vi "Reset Window.vi"(8 "error in (no error)":errorcluster, 11 "Rigol DG822 Sine in":refnum<class "Rigol DG822 Sine.lvclass">) -> (0 "error out":errorcluster, 3 "Rigol DG822 Sine out":refnum<class "Rigol DG822 Sine.lvclass">)   [LabVIEW 2021, in "Rigol DG822 UI.lvlib" / "Rigol DG822 Sine.lvlib" / "Rigol DG822 Sine.lvclass"]
uses:
  Rigol DG822 Sine.lvclass
  General/Files/lvlibp/Actors.lvlibp/Actors/Actors/Actors.lvclass
  D:/LabVIEW/General/Files/lvlibp/Actors.lvlibp/Actors/Actors/Actors.lvclass
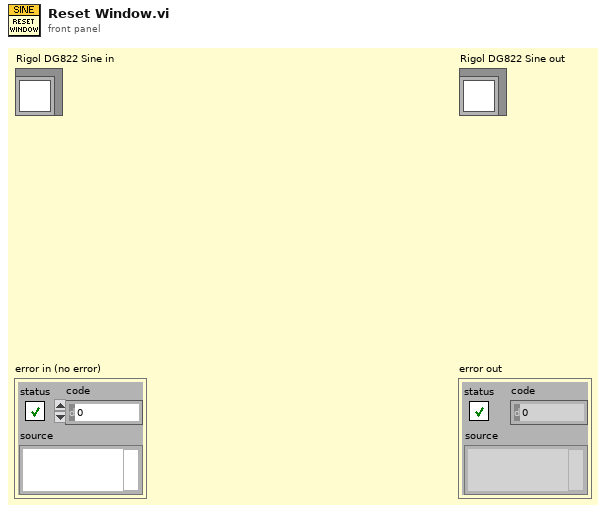
[diagram p1: front panel]
types:
  T1 = cluster{"Control Label 5":string, "Control Label 6":string, "Control Label":string, "Control Label 2":string, "Control Label 3":string, "Control Label 4":string}
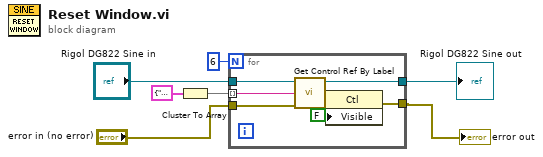
[diagram p0: block diagram]
diagram:
  n1 = Cluster To Array(cluster=T1 {"Control Label 5"="FreqUnit", "Control Label 6"="PeriodUnit", "Control Label"="AmplUnit", "Control Label 2"="HighLUnit", "Control Label 3"="OffsetUnit", "Control Label 4"="LowLUnit"}) -> (array=w6:string[])
  n2 = for {
    N: 6 -> [_]
    tunnel: [w12] -> w1
    tunnel: "Rigol DG822 Sine in" -> [w11]
    tunnel: w6 -> [w10] mode=indexing
    tunnel: "error in (no error)" -> [w9]
    tunnel: [w8] -> w2
    n3 = call "Get Control Ref By Label.vi"("error in (no error)"=w9, "Control Label"=w10, "Actors in"=w11) -> ("error out"=w14:errorcluster, "Control Ref"=w13:refnum<vi>, "Actors out"=w12:refnum<class "Rigol DG822 Sine.lvclass">)  [unwired: 6 in]
    n4 = property class="Ctl"(reference=w13, error in=w14, "Visible"=FALSE) -> (error out=w8:errorcluster)  [unwired: 1 out]
  }
  "error out" <- w2
  "Rigol DG822 Sine out" <- w1
